vi "load system from file data.vi"(8 "error in":errorcluster, 11 "file information":T4) -> (0 "error out":errorcluster, 3 "system":T1)   [LabVIEW 2013, in "PLConfigurationSerializer.lvlib"]
uses:
  PLConfigurationSerializer.lvlib
  1_0_0_0 format.ctl
  system hierarchy.ctl
  target hierarchy.ctl
  engine hierarchy.ctl
  configuration database.ctl
  systems cluster.ctl
  system configuration/PL_System Configuration.lvclass
  targets cluster.ctl
  target configuration/PL_Target Configuration.lvclass
  engines cluster.ctl
  <vilib>/NI/Module Execution Interface/Engine Configuration/engine configuration.lvclass
  <vilib>/NI/Tag Bus Module Framework/module configuration/TBM module configuration.lvclass
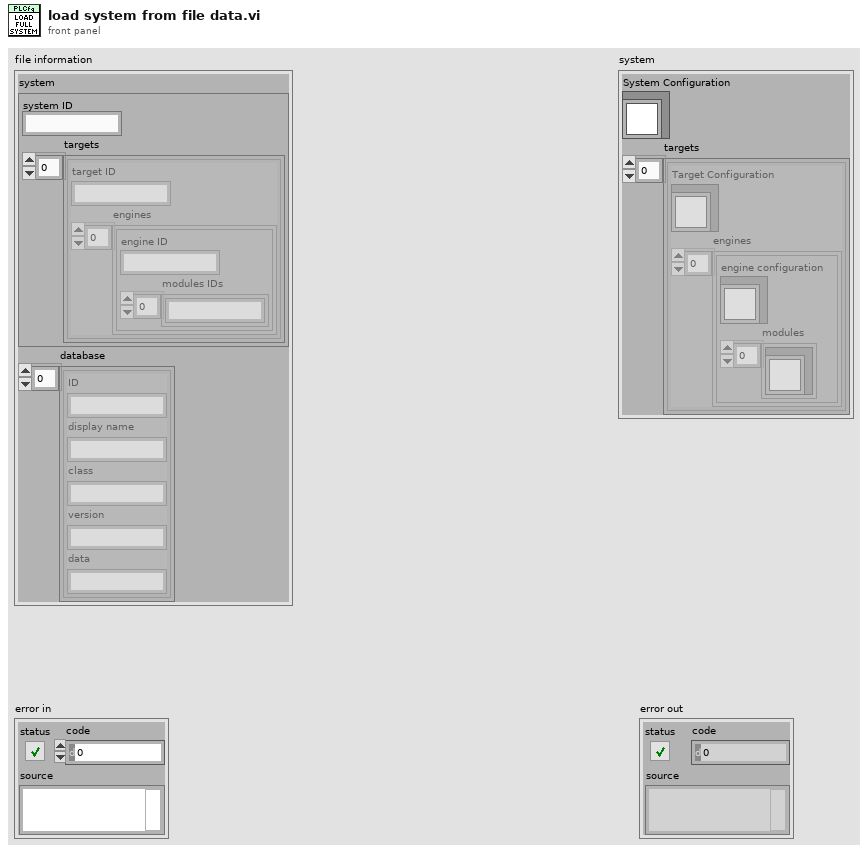
[diagram p1: front panel]
types:
  T1 = typedef "PLConfigurationSerializer.lvlib/systems cluster.ctl" = cluster{"System Configuration":refnum<class "PL_System Configuration.lvclass">, "targets":T2[]}
  T2 = typedef "PLConfigurationSerializer.lvlib/targets cluster.ctl" = cluster{"Target Configuration":refnum<class "PL_Target Configuration.lvclass">, "engines":T3[]}
  T3 = typedef "PLConfigurationSerializer.lvlib/engines cluster.ctl" = cluster{"engine configuration":refnum<class "engine configuration.lvclass">, "modules":refnum<class "TBM module configuration.lvclass">[]}
  T4 = typedef "PLConfigurationSerializer.lvlib/1_0_0_0 format.ctl" = cluster{"system":T5, "database":T8[]}
  T5 = typedef "PLConfigurationSerializer.lvlib/system hierarchy.ctl" = cluster{"system ID":string, "targets":T6[]}
  T6 = typedef "PLConfigurationSerializer.lvlib/target hierarchy.ctl" = cluster{"target ID":string, "engines":T7[]}
  T7 = typedef "PLConfigurationSerializer.lvlib/engine hierarchy.ctl" = cluster{"engine ID":string, "modules IDs":string[]}
  T8 = typedef "PLConfigurationSerializer.lvlib/configuration database.ctl" = cluster{"ID":string, "display name":string, "class":string, "version":string, "data":string}
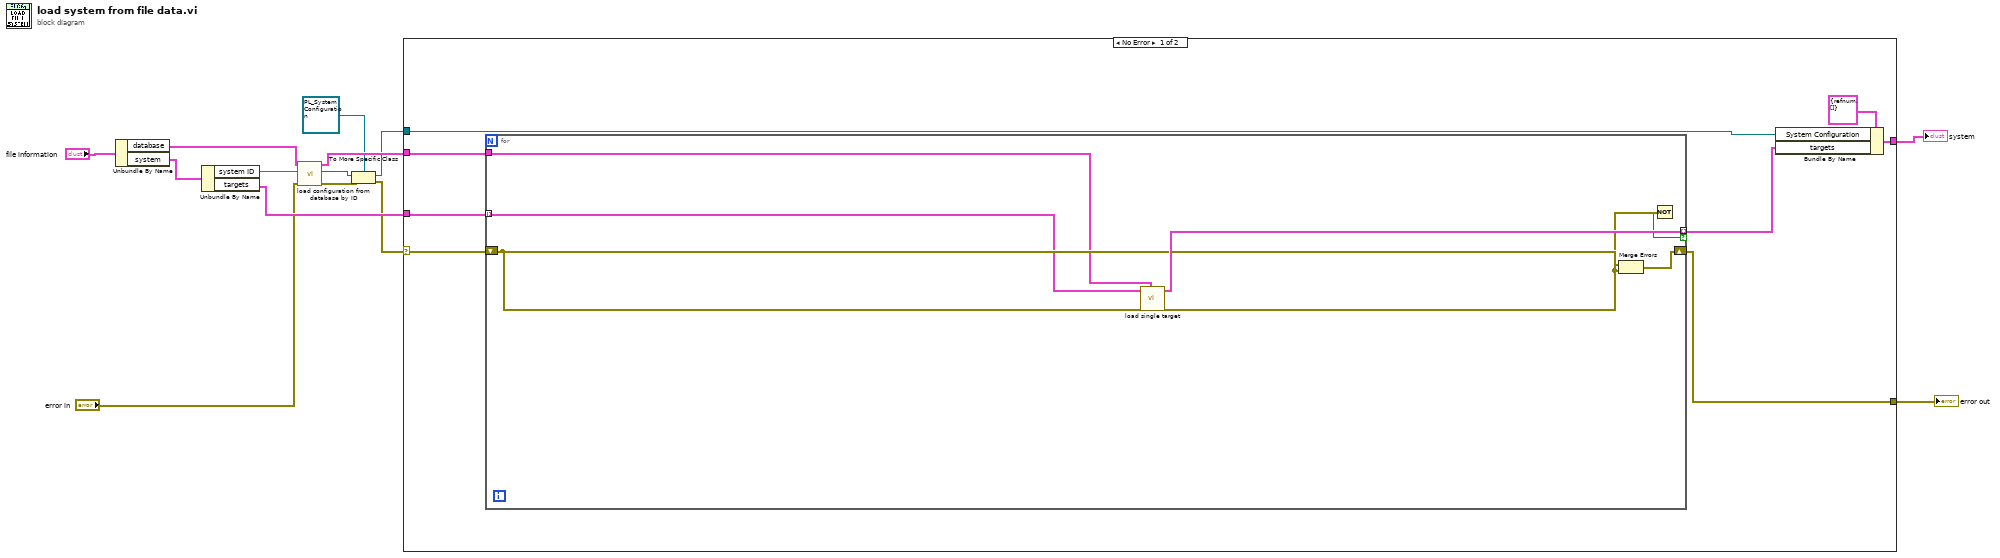
[diagram p0: block diagram]
diagram:
  n1 = Unbundle By Name("file information") -> ("database"=w10:T8[], "system"=w12:T5)
  n2 = Unbundle By Name(w12) -> ("system ID"=w7:string, "targets"=w11:T6[])
  n3 = call "load configuration from database by ID.vi"("error in"="error in", "ID"=w7, "database in"=w10) -> ("error out"=w6:errorcluster, "configuration"=w5:refnum<class "TBM configuration.lvclass">, "database out"=w9:T8[])  [unwired: 6 in]
  n4 = To More Specific Class(target class=refnum<class "PL_System Configuration.lvclass"> refnum ("System Configuration"), reference=w5, error in=w6) -> (specific class reference=w3:refnum<class "PL_System Configuration.lvclass">, error out=w2:errorcluster)
  n5 = case shown="No Error" w2 {
    selector: w2 -> [w16 w30]
    tunnel: [w21 _] -> w14
    tunnel: w11 -> [w20 _]
    tunnel: w9 -> [w18 _]
    tunnel: w3 -> [w17 _]
    tunnel: [w15 w30] -> w1
    frame No Error {
      n6 = for {
        tunnel: w20 -> [w23] mode=indexing
        tunnel: [w29] -> w19 mode=indexing if=w25
        shift-right: [w27] -> w15
        shift-left: w16 -> [w28]
        tunnel: w18 -> [w24]
        n7 = call "load single target.vi"("database in"=w24, "error in"=w28, "target to load"=w23) -> ("error out"=w26:errorcluster, "targets cluster out"=w29:T2)  [unwired: 7 in]
        n8 = Merge Errors(w28, w26) -> (w27:errorcluster)
        n9 = Not(x=w26) -> (.not. x?=w25:bool)
      }
      n10 = Bundle By Name(cluster=T1 {"System Configuration"=refnum, "targets"=[]} ("system"), "System Configuration"=w17, "targets"=w19) -> (w21:T1)
    }
    frame Error {
    }
  }
  "system" <- w14
  "error out" <- w1
